vi "dataHandler_pend_fw3.vi"() -> ()   [LabVIEW 2022 SP3]
uses:
  LVLib/SADI_FW3.lvlib
panel:
  in  "instance":i32
  in  "pendMotorVal":u16 max=1023
  in  "pendDir":bool=TRUE
  out "Pendulum ENC":u16
  out "MSG CNT":u32
  out "ENC VEL 0":u16
  out "ENC POS 0":i32
  in  "Latest?":bool=TRUE
  in  "enableWrite":bool=TRUE
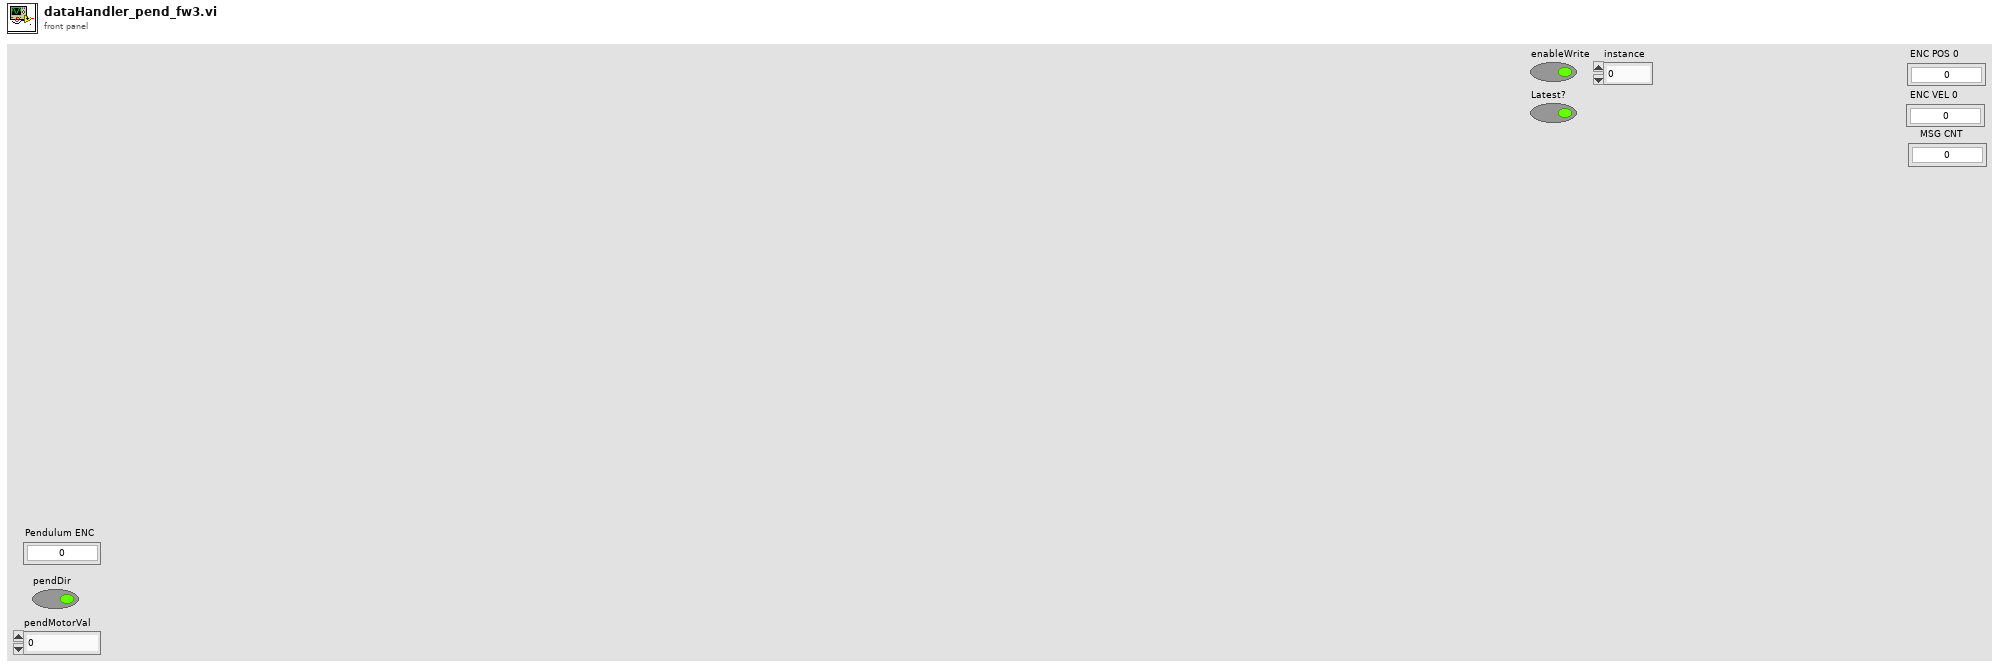
[diagram p1: front panel]
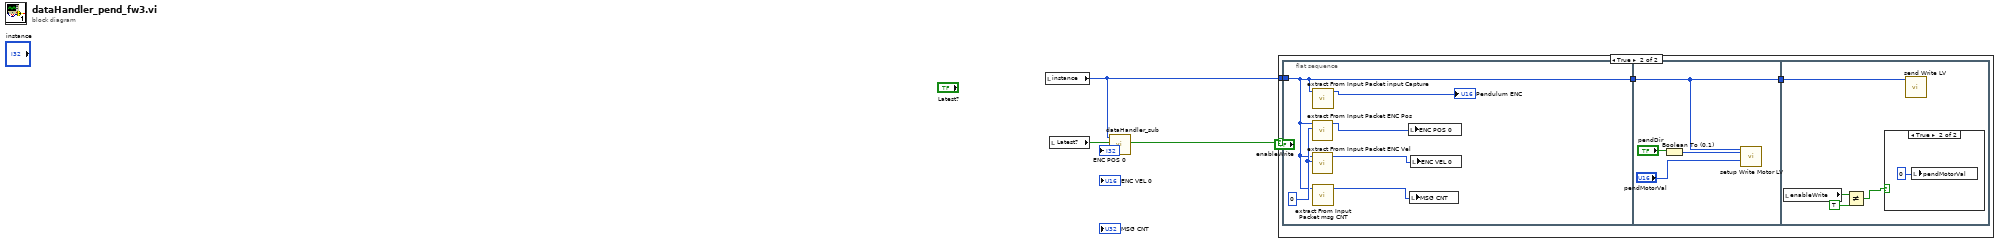
[diagram p0: block diagram]
diagram:
  n1 = local read "instance"() -> (w1:i32)
  n2 = local read "Latest?"() -> (w2:bool)
  n3 = call "dataHandler_sub.vi"("Instance"=w1, "Latest?"=w2) -> ("dataToRead?"=w3:bool)  [unwired: 7 in, 1 out]
  n4 = case shown="True" w3 {
    tunnel: w1 -> [_ w6]
    frame False {
    }
    frame True {
      n5 = flat-sequence {
        tunnel: w6 -> [w8]
        tunnel: [w8] -> w5
        tunnel: w5 -> [w15]
        tunnel: [w15] -> w4
        tunnel: w4 -> [w20]
        frame #0 {
          w12 = 0 ("channel")
          n6 = call "extract From Input Packet ENC Pos.vi"("channel"=w12, "instance"=w8) -> ("function return"=w11:i32)  [unwired: 9 in]
          n7 = call "extract From Input Packet ENC Vel.vi"("channel"=w12, "instance"=w8) -> ("function return"=w10:u16)  [unwired: 9 in]
          n8 = call "extract From Input Packet input Capture.vi"("instance"=w8) -> ("function return"=→"Pendulum ENC":u16)  [unwired: 10 in]
          n9 = call "extract From Input Packet msg CNT.vi"("instance"=w8) -> ("function return"=w9:u32)  [unwired: 10 in]
          n10 = local write "ENC POS 0"(w11) -> ()
          n11 = local write "MSG CNT"(w9) -> ()
          n12 = local write "ENC VEL 0"(w10) -> ()
        }
        frame #1 {
          n13 = Boolean To (0,1)(Boolean="pendDir") -> (0, 1=w13:i16)
          n14 = call "setup Write Motor LV.vi"("value"="pendMotorVal", "motorNum"=w13, "instance"=w15) -> ()  [unwired: 9 in]
        }
        frame #2 {
          n15 = local read "enableWrite"() -> (w19:bool)
          n16 = Not Equal?(x=w19, y=TRUE) -> (x != y?=w17:bool)
          n17 = case shown="True" w17 {
            frame False {
            }
            frame True {
              n18 = local write "pendMotorVal"(u16 0 ("pendMotorVal")) -> ()
            }
          }
          n19 = call "send Write LV.vi"("instance"=w20) -> ()  [unwired: 11 in]
        }
      }
    }
  }
